vi "Co-Pilot Loop.vi"(11 "Co_fifo":refnum<k33>) -> ()   [LabVIEW 2014]
uses:
  Co-Pilot_game_control.ctl
  MechanismMetrics.ctl
  Lifter States.ctl
  Auto Lifter States.ctl
  <vilib>/Platform/TimedLoop/XDataNode/timing_clust.ctl
  <vilib>/Platform/TimedLoop/XDataNode/nitl_modes.ctl
  <vilib>/Platform/TimedLoop/XDataNode/wakeup.ctl
  <vilib>/platform/TimedLoop/XDataNode/XDataNode.xnode
  <vilib>/Platform/TimedLoop/XDataNode/XDNodeRunTimeDep.lvlib
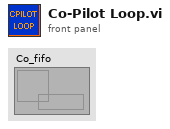
[diagram p1: front panel]
types:
  T1 = typedef "MechanismMetrics.ctl" = cluster{"lift height":dbl, "Command":enum16{"Noop", "Flagged"}, "Time Stamp":u32, "ToggleCollector":bool, "Bottom_Limit_Switch ":bool, "Top_Limit_Switch":bool, "lift power":dbl, "Elevator soleniod debounce time   ":dbl, "LifterOverride":bool, "Previous Lift power":dbl, "manual lift":dbl, "Lifter State":T2, "Auto Lifter State":T3, "Toggle Auto Lifter":bool, "Wait Timer":dbl, "HP Auto Indexer":bool, "HP Auto Lifter State":T3, "Commanded Velocity":dbl, "\nActive collect":dbl, "CG Teleop":bool}
  T2 = typedef "Lifter States.ctl" = enum16{"OpeningLifter", "LifterOpen", "ClosingLifter", "LifterClosed"}
  T3 = typedef "Auto Lifter States.ctl" = enum16{"Not Pressed", "THE_END", "WAIT_FOR_RELEASE", "Press Detected", "To Release Stacked1", "To Collect", "Open Lifter", "WAIT", "Close", "To Stack1"}
  T4 = typedef "XDNodeRunTimeDep.lvlib/timing_clust.ctl" = cluster{"Expected End [f-1]":u64, "Actual End [f-1]":u64, "Finished Late? [f-1]":bool, "Expected End [i-1]":u64, "Actual End [i-1]":u64, "Finished Late? [i-1]":bool, "Expected Start [i]":u64, "Actual Start [i]":u64, "Expected Start [f]":u64, "Actual Start [f]":u64, "Source Name":string, "Structure Name":string, "Period":i64, "Deadline":i64, "Offset":i64, "Start":i64, "Priority":i32, "Timeout":i32, "Mode":T5, "Wakeup Reason":T6, "Error":errorcluster, "Source Type":string, "Secondary Source Type":string, "Global End Time":u64, "Global Start Time":u64, "Frame Duration":u64, "Iteration Duration":u64, "Assigned CPU":i32, "I/O Scan Engine Mode":u32}
  T5 = typedef "XDNodeRunTimeDep.lvlib/nitl_modes.ctl" = enum32{"No Change", "Process missed periods, maintain original phase", "Discard missed periods, maintain original phase", "Process missed periods, ignore original phase", "Discard missed periods, ignore original phase"}
  T6 = typedef "XDNodeRunTimeDep.lvlib/wakeup.ctl" = enum32{"Normal", "Aborted", "Asynchronous wakeup", "Timing source error", "Timed loop error", "Timeout"}
  T7 = typedef "Co-Pilot_game_control.ctl" = cluster{"Left_Intake":dbl, "Right_Intake":dbl, "Time Stamp":u32, "Command":enum16{"Noop", "Flagged"}, "ToggleCollector":bool, "ManualLift":dbl, "Top_Limit_Switch":bool, "Bottom_Limit_Switch ":bool, "LifterOverride":bool, "AutoLift":i32, "Toggle Auto Lifter":bool, "Activate HP indexer":bool, "CGTeleopButton":bool}
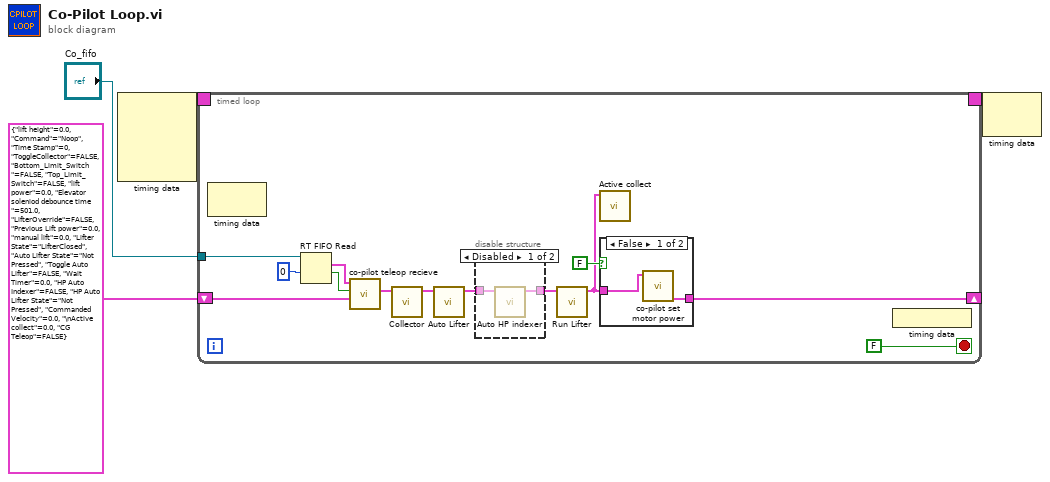
[diagram p0: block diagram]
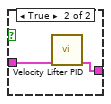
[diagram p2: hidden frame]
diagram:
  n1 = node-c288() -> (w4:T4)  [unwired: 4 in]
  n2 = timed-loop {
    timing: w4 -> [_]
    timing-out: [_] -> w3
    tunnel: "Co_fifo" -> [w16]
    shift-right: [w5] -> _
    shift-left: T1 {"lift height"=0.0, "Command"=enum."Noop", "Time Stamp"=0, "ToggleCollector"=FALSE, "Bottom_Limit_Switch "=FALSE, "Top_Limit_Switch"=FALSE, "lift power"=0.0, "Elevator soleniod debounce time   "=501.0, "LifterOverride"=FALSE, "Previous Lift power"=0.0, "manual lift"=0.0, "Lifter State"=enum."LifterClosed", "Auto Lifter State"=enum."Not Pressed", "Toggle Auto Lifter"=FALSE, "Wait Timer"=0.0, "HP Auto Indexer"=FALSE, "HP Auto Lifter State"=enum."Not Pressed", "Commanded Velocity"=0.0, "\nActive collect"=0.0, "CG Teleop"=FALSE} ("MechanismMetrics") -> [w12]
    stop <- FALSE stop-if-true
    n3 = node-c288() -> ()  [unwired: 1 in, 1 out]
    n4 = RT FIFO Read(0:w16, 2:0 ("timeout in ms (0)")) -> (9:w15:T7, 10:w13:bool)  [unwired: 2 in, 3 out]
    n5 = call "co-pilot teleop recieve.vi"("MechanismMetrics in"=w12, "empty?"=w13, "Co-Pilot Data in"=w15) -> ("MechanismMetrics out"=w11:T1)  [unwired: 8 in]
    n6 = call "Collector.vi"("MechanismMetrics in"=w11) -> ("MechanismMetrics out"=w10:T1)  [unwired: 10 in]
    n7 = call "Auto Lifter.vi"("MechanismMetrics in"=w10) -> ("MechanismMetrics in 2"=w9:T1)  [unwired: 10 in]
    n8 = disable-structure shown="Disabled" {
      disable-tunnel: w9 -> [w23 w24]
      disable-tunnel: [w22 w24] -> w8
      frame Disabled {
        n9 = call "Auto HP indexer.vi"("MechanismMetrics in"=w23) -> ("MechanismMetrics in 2"=w22:T1)  [unwired: 10 in]
      }
      frame Enabled {
      }
    }
    n10 = call "Run Lifter.vi"("MechanismMetrics in"=w8) -> ("MechanismMetrics out"=w6:T1)  [unwired: 10 in]
    n11 = call "Active collect.vi"("MechanismMetrics in"=w6) -> ()  [unwired: 11 in]
    n12 = case shown="False" FALSE {
      tunnel: [w19 w21] -> w5
      tunnel: w6 -> [w18 w20]
      frame False {
        n13 = call "co-pilot set motor power.vi"("MechanismMetrics"=w18) -> ("MechanismMetrics 2"=w19:T1)  [unwired: 9 in, 1 out]
      }
      frame True {
        n14 = call "Velocity Lifter PID.vi"("MechanismMetrics"=w20) -> ("MechanismMetrics 2"=w21:T1)  [unwired: 10 in]
      }
    }
    n15 = node-c288() -> ()  [unwired: 1 out]
  }
  n16 = node-c288(w3) -> ()  [unwired: 1 out]
